vi "Area of Triangle.vi"(1 "Side C (cm)":dbl, 2 "Side B (cm)":dbl, 3 "Side A (cm)":dbl) -> (0 "Area of Triangle (cm^2)":dbl)   [LabVIEW 2015]
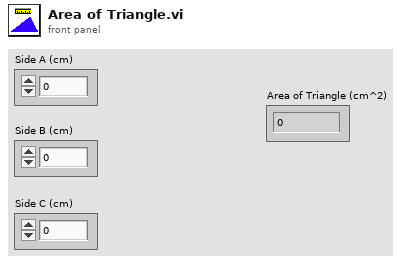
[diagram p1: front panel]
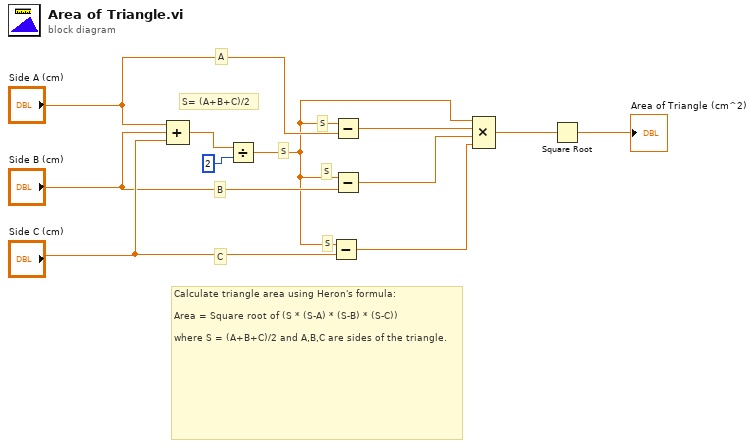
[diagram p0: block diagram]
diagram:
  # "A"
  # "B"
  # "C"
  # "S"
  # "S"
  # "S"
  # "S"
  # "S= (A+B+C)/2"
  # "Calculate triangle area using Heron's formula:\n\nArea = Square root of (S * (S-A) * (S-B) * (S-C))\n\nwhere S = (A+B+C)/2 and A,B,C are sides of the triangle."
  n1 = Compound Arithmetic op=ADD("Side A (cm)", "Side B (cm)", "Side C (cm)") -> (w5:dbl)
  n2 = Divide(x=w5, y=2) -> (x/y=w1:dbl)
  n3 = Subtract(x=w1, y="Side C (cm)") -> (x-y=w8:dbl)
  n4 = Subtract(x=w1, y="Side A (cm)") -> (x-y=w10:dbl)
  n5 = Subtract(x=w1, y="Side B (cm)") -> (x-y=w9:dbl)
  n6 = Compound Arithmetic op=MULTIPLY(w1, w10, w9, w8) -> (w7:dbl)
  n7 = Square Root(x=w7) -> (sqrt(x)=→"Area of Triangle (cm^2)":dbl)
